vi "niRFUtil WFM Create Waveform Mask.vi"(2 "Waveform In":T1 {"y" min=0 max=127 format="%.2f"; "dx" format="%^.2e"; "x0" format="%^.2e"}, 3 "Mask":cluster{"Time, sec":dbl[], "Mask Value":sgl[]} {"Mask Value" format="%.2f"; "Time, sec" format="%^.2e"}) -> (1 "Mask Points":T1 {"y" min=0 max=127 format="%.2f"; "dx" format="%^.2e"; "x0" format="%^.2e"})   [LabVIEW 2015, in "niRFUtil.lvlib"]
doc: "(c) Copyright 2006, National Instruments, Inc. This VI may not be duplicated, sold, or distributed without written consent from National Instruments."
uses:
  niRFUtil.lvlib
  Includes/niRFUtil INC Real Waveform.ctl
  Includes/niRFUtil INC Real Array.ctl
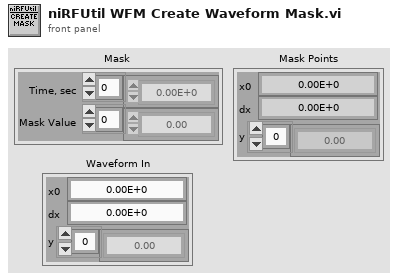
[diagram p1: front panel]
types:
  T1 = typedef "niRFUtil.lvlib/niRFUtil INC Real Waveform.ctl" = cluster{"x0":dbl, "dx":dbl, "y":T2}
  T2 = typedef "niRFUtil.lvlib/niRFUtil INC Real Array.ctl" = sgl[]
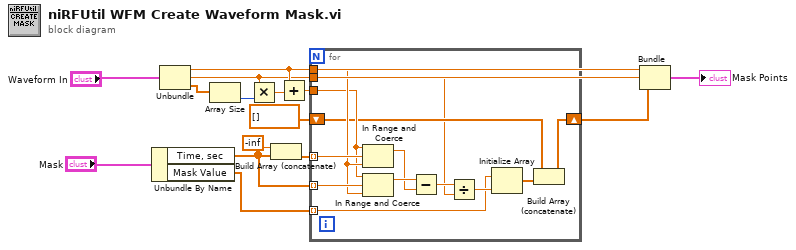
[diagram p0: block diagram]
diagram:
  n1 = Unbundle By Name("Mask") -> ("Time, sec"=w5:dbl[], "Mask Value"=w6:sgl[])
  n2 = Unbundle("Waveform In") -> ("x0"=w9:dbl, "dx"=w7:dbl, "y"=w12:T2)
  n3 = Array Size(array=w12) -> (size(s)=w11:i32)
  n4 = Multiply(x=w7, y=w11) -> (x*y=w10:dbl)
  n5 = Build Array (concatenate)(-inf, w5) -> (w4:dbl[])
  n6 = Add(x=w9, y=w10) -> (x+y=w8:dbl)
  n7 = for {
    tunnel: w4 -> [w28] mode=indexing
    shift-right: [w19] -> w14
    shift-left: sgl[] [] ("y") -> [w20]
    tunnel: w9 -> [w26]
    tunnel: w8 -> [w25]
    tunnel: w5 -> [w27] mode=indexing
    tunnel: w7 -> [w16]
    tunnel: w6 -> [w21] mode=indexing
    n8 = In Range and Coerce(upper limit=w25, x=w28, lower limit=w26) -> (coerced(x)=w23:dbl)  [unwired: 1 out]
    n9 = In Range and Coerce(upper limit=w25, x=w27, lower limit=w26) -> (coerced(x)=w24:dbl)  [unwired: 1 out]
    n10 = Subtract(x=w24, y=w23) -> (x-y=w17:dbl)
    n11 = Divide(x=w17, y=w16) -> (x/y=w22:dbl)
    n12 = Initialize Array(w21, w22) -> (w18:sgl[])
    n13 = Build Array (concatenate)(w20, w18) -> (w19:sgl[])
  }
  n14 = Bundle("x0"=w9, "dx"=w7, "y"=w14) -> (→"Mask Points":cluster{"x0":dbl, "dx":dbl, "y":sgl[]})  [unwired: 1 out]
